vi "Draw Color Frame.vi"(8 "Error In":errorcluster, 10 "U32 Array":u8[](array[numeric]), 11 "Image":T1) -> (0 "Error Out":errorcluster, 3 "Image Out":T1)   [LabVIEW 2011, in "KinectOne.lvlib"]
doc: "Converts the Color data to an RGB U32 IMAQ Image."
uses:
  KinectOne.lvlib
  <vilib>/vision/Image Controls.llb/IMAQ Image.ctl
  Private/Frame Description FGV [Color].vi
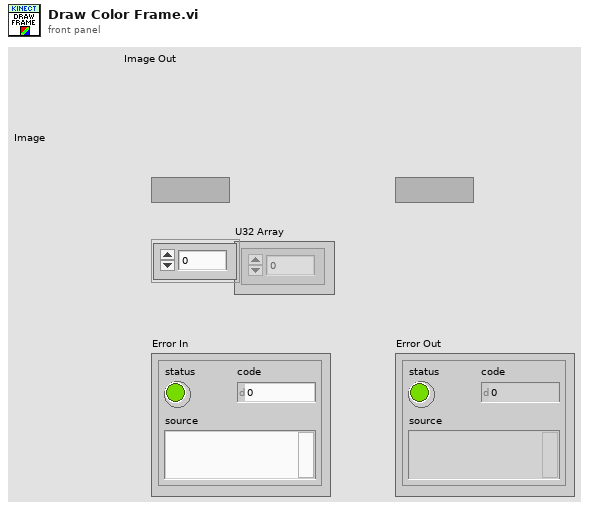
[diagram p1: front panel]
types:
  T1 = typedef "IMAQ Image.ctl" = refnum<image>
  T2 = typedef "KinectOne.lvlib/FrameDescription.ctl" = cluster{"BytesPerPixel":u32, "DiagonalFieldOfView":sgl, "Height":i32, "HorizontalFieldOfView":sgl, "LengthInPixels":u32, "VerticalFieldOfView":sgl, "Width":i32}
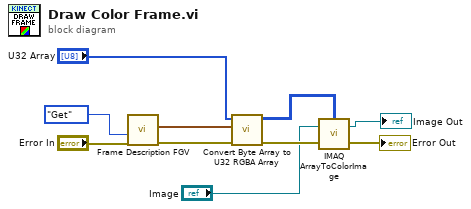
[diagram p0: block diagram]
diagram:
  n1 = call-poly "Frame Description FGV.vi"("error in (no error)"="Error In", "Command"=enum16{"Get", "Set"}."Get") -> ("error out"=w6:errorcluster, "FrameDescription"=w5:T2)  [unwired: 8 in]
  n2 = call "Convert Byte Array to U32 RGBA Array.vi"("error in (no error)"=w6, "FrameDescription"=w5, "Byte Array"="U32 Array") -> ("error out"=w10:errorcluster, "RGBA U32 Array"=w9:u32[][])  [unwired: 7 in]
  n3 = call "IMAQ ArrayToColorImage"("Image Pixels (U32)"=w9, "Image"="Image", "error in (no error)"=w10) -> ("Image Out"=→"Image Out":T1, "error out"=→"Error Out":errorcluster)  [unwired: 2 in]
